vi "ROTPEN Control template CLEAN.vi"() -> ()   [LabVIEW 2018]
uses:
  <vilib>/Simulation/Scripting/Companion Diagram/SimConfigNode/SimParams.ctl
  <vilib>/Simulation/Scripting/Companion Diagram/SimConfigNode/_simSolvers.ctl
  <vilib>/Simulation/Implementation/Shared/SIMSCR Execution Mode.ctl
  <vilib>/Platform/TimedLoop/XDataNode/timing_clust.ctl
  <vilib>/Platform/TimedLoop/XDataNode/nitl_modes.ctl
  <vilib>/Platform/TimedLoop/XDataNode/wakeup.ctl
  <vilib>/Simulation/Param Hierarchy/Typedefs/SIMPH Param Control Actions.ctl
  <vilib>/addons/Control Design/_Stochastic Systems/Stochastic Systems.llb/Stochastic Systems SubVIs/cd_Second-Order Statistics Noise Model.ctl
  <vilib>/Simulation/Scripting/Editor Utilities/SIM subVI tag data.ctl
  <vilib>/Simulation/Scripting/Editor Utilities/SIM subVI execution type.ctl
  <vilib>/Simulation/Implementation/Shared/NILVSim_ParamChanged.vi
  <vilib>/Simulation/Implementation/Shared/NILVSim_FinishedLate.vi
  <vilib>/Simulation/Implementation/Shared/NILVSIM_BeginStep.vi
  <vilib>/Simulation/DataSources/Implementation/NILVSim Signal Generator.llb/SIM Signal Generator (scalar).vi
  <vilib>/Simulation/SignalArithmetic/Implementation/NILVSim Gain.llb/SIM Gain (scalar).vi
  <vilib>/Simulation/Utility/Implementation/SIM Halt.vi
  <vilib>/Simulation/ContinuousLinear/Implementation/NILVSim Derivative.llb/SIM derivative (scalar).vi
  <vilib>/Simulation/SignalArithmetic/Implementation/NILVSim Gain.llb/SIM Gain (vector,ScalarGain).vi
  <vilib>/Simulation/SignalArithmetic/Implementation/NILVSim Gain.llb/SIM Gain (dot product).vi
  <vilib>/Simulation/Nonlinear/Implementation/NILVSim Saturation.llb/SIM Saturation (scalar).vi
  <vilib>/Simulation/Implementation/Shared/SIM Fire Discrete SubVI.vi
  <vilib>/Simulation/Implementation/Shared/NILVSim_Manager.vi
  <vilib>/Utility/error.llb/Clear Errors.vi
  <vilib>/Simulation/Implementation/Shared/NILVSim_FinalizeModel.vi
  <vilib>/Simulation/Implementation/Shared/SIM Fire Discrete SubVI (Core).vi
  <vilib>/addons/Control Design/_Stochastic Systems/Stochastic Systems.llb/CD Construct Stochastic Model (Numeric).vi
  <vilib>/addons/Control Design/_Stochastic Systems/Stochastic Systems.llb/CD Construct Noise Model (Numeric).vi
  <vilib>/Simulation/Implementation/Shared/SIM Unbundle Sim Info.vi
  <vilib>/Simulation/Implementation/Shared/SIMSH Read Queue.vi
  <vilib>/Simulation/Implementation/Shared/NILVSim_Initialize.vi
  <vilib>/Simulation/Utility/Implementation/NILVSim Get Time and IsAcceptedStep.vi
  <vilib>/Simulation/Implementation/Shared/NILVSim_GetModelError.vi
  <vilib>/Simulation/Implementation/Shared/SIM Bundle Sim Info.vi
  <vilib>/Simulation/Scripting/Companion Diagram/SimConfigNode/SimDog.xnode
  <vilib>/Quanser/Rapid Control Prototyping Toolkit/hardware/HIL Immediate IO/_TypeSpecific/CL HIL Read Encoder (Vector).vi
  <vilib>/Quanser/Rapid Control Prototyping Toolkit/hardware/HIL Immediate IO/CL HIL Read.vi
  <vilib>/Quanser/Rapid Control Prototyping Toolkit/hardware/HIL Immediate IO/_TypeSpecific/CL HIL Write Analog (Scalar).vi
  <vilib>/Quanser/Rapid Control Prototyping Toolkit/hardware/HIL Immediate IO/CL HIL Write.vi
  <vilib>/addons/Control Design/_Implementation/CD Continuous Recursive Kalman Filter.vi
  <vilib>/Platform/TimedLoop/XDataNode/XDataNode.xnode
  <vilib>/Simulation/Implementation/XNodeFramework/SimXNode/SimX.xnode
  <vilib>/addons/Control Design/_Stochastic Systems/NI_CD_Stochastic Systems.lvlib
  <vilib>/Platform/TimedLoop/XDataNode/XDNodeRunTimeDep.lvlib
  <vilib>/Simulation/Implementation/Shared/NI_SIM_Implementation.lvlib
panel:
  out "Encoder Velocities (Kalman)":T1(graph)
  out "Encoder Angles (Kalman)":T1(graph)
  in  "stop":bool
  out "Motor Voltage (V)":dbl(graph)
  out "Encoder Angles (deg)":T2(graph)
  out "Encoder Velcoities (deg)":T3(graph)
  in  "Frequency (Hz)":dbl(slide)=0.2 min=0.0 max=0.5 step=0.05 scale=0.0..0.5 scale format="%#_3f"
  in  "Amplitude (deg)":dbl(slide) min=0.0 max=40.0 step=5.0 scale=0.0..40.0
  # "Rotary Arm Reference Signal"
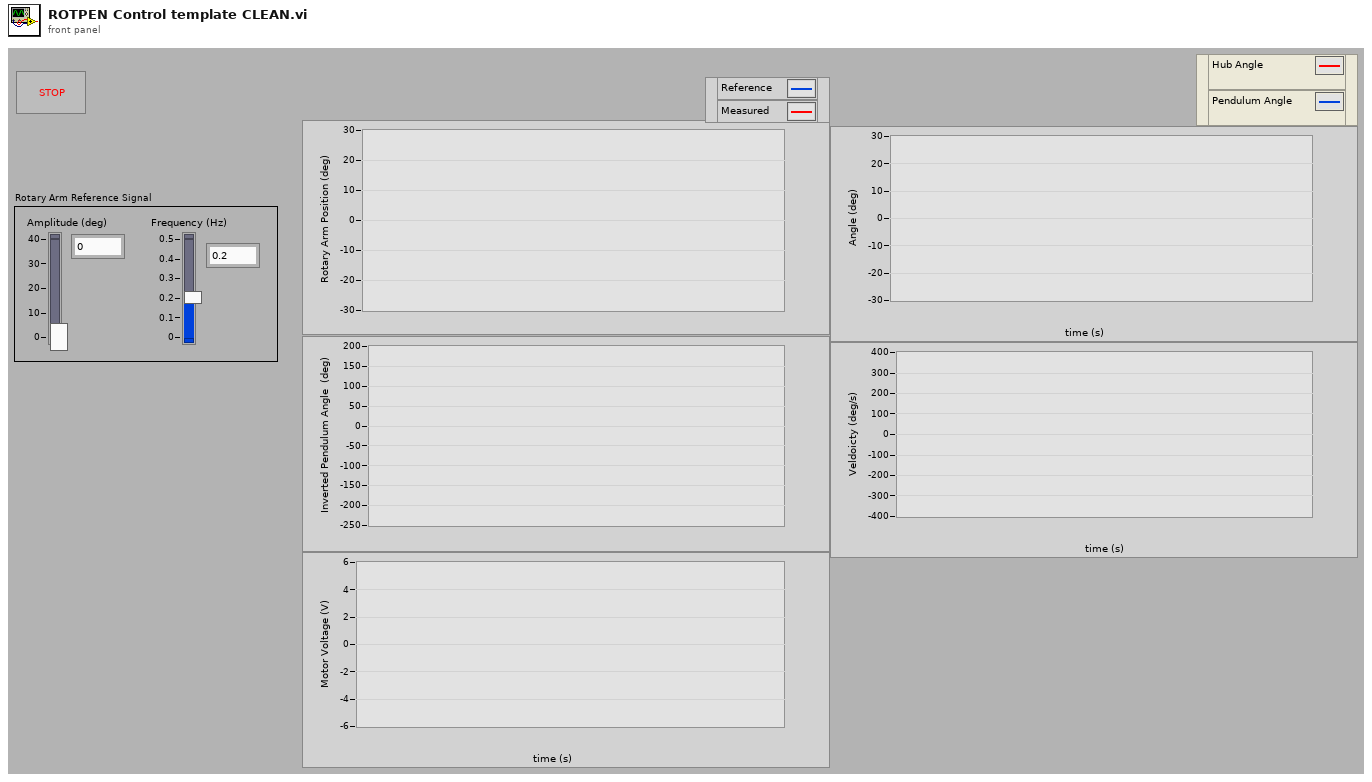
[diagram p1: front panel]
types:
  T1 = cluster{"Estimated State xhat(t)[0]":dbl, "Estimated State xhat(t)[1]":dbl, "Estimated State xhat(t)[2]":dbl, "Estimated State xhat(t)[3]":dbl, "Estimated State xhat(t)[4]":dbl, "Estimated State xhat(t)[5]":dbl, "Estimated State xhat(t)[6]":dbl, "Estimated State xhat(t)[7]":dbl, "Estimated State xhat(t)[8]":dbl}
  T2 = cluster{"output":dbl, "output":dbl, "output":dbl}
  T3 = cluster{"output[0]":dbl, "output[1]":dbl, "output[2]":dbl, "output[3]":dbl, "output[4]":dbl, "output[5]":dbl, "output[6]":dbl, "output[7]":dbl, "output[8]":dbl}
  T4 = typedef "NI_CD_Stochastic Systems.lvlib/cd_Stochastic State-Space Model.ctl" = cluster{"Sampling Time (s)":dbl, "G":dbl[][], "B":dbl[][], "A":dbl[][], "C":dbl[][], "D":dbl[][], "H":dbl[][]}
  T5 = typedef "NI_CD_Stochastic Systems.lvlib/cd_Second-Order Statistics Noise Model.ctl" = cluster{"Q":dbl[][], "E{w}":dbl[], "E{v}":dbl[], "R":dbl[][], "N":dbl[][]}
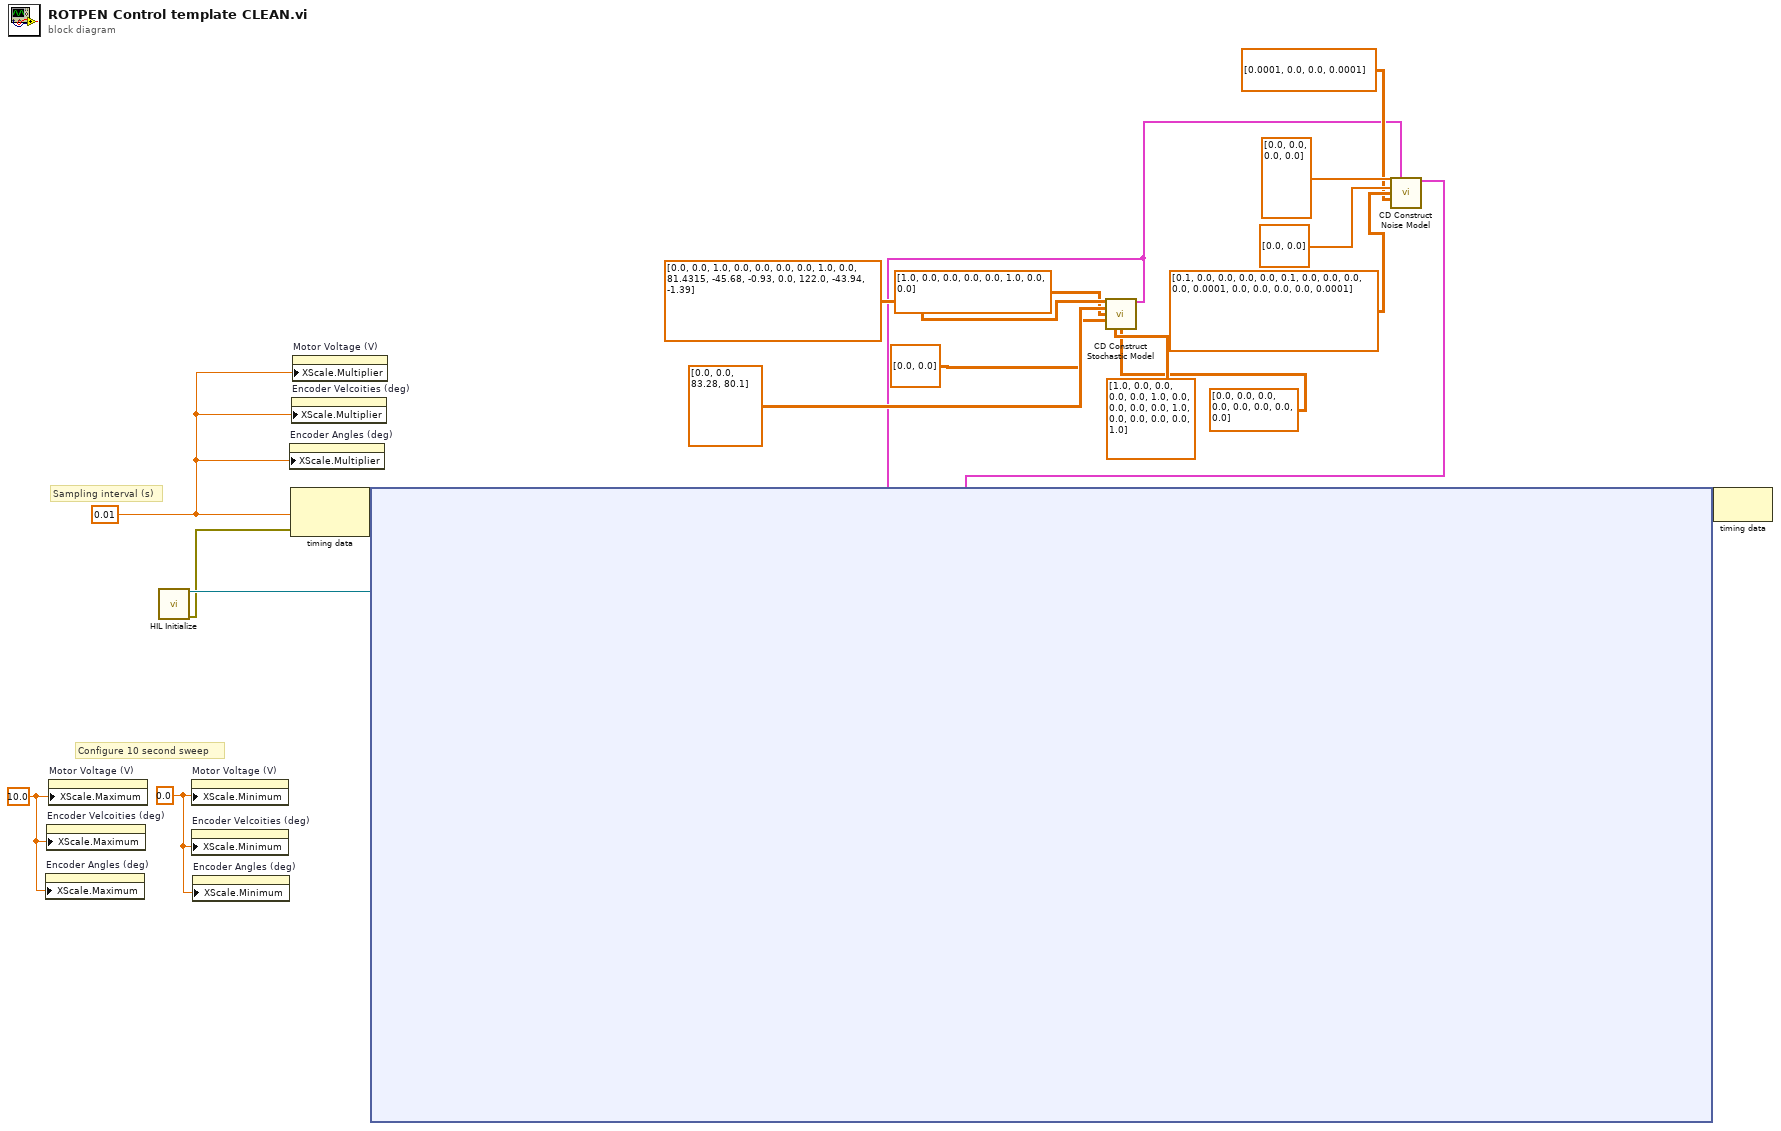
[diagram p0: block diagram]
diagram:
  w15 = 0.0 ("X Scale.Range:Maximum")
  w14 = 10.0 ("X Scale.Range:Maximum")
  w2 = 0.01 ("Step Size (s)")
  # "Configure 10 second sweep"
  # "Sampling interval (s)"
  n1 = property on="Encoder Angles (deg)" class="WFChart (strict)"("XScale.Maximum"=w14) -> ()  [unwired: 2 in, 2 out]
  n2 = property on="Encoder Velcoities (deg)" class="WFChart (strict)"("XScale.Maximum"=w14) -> ()  [unwired: 2 in, 2 out]
  n3 = property on="Motor Voltage (V)" class="WFChart (strict)"("XScale.Maximum"=w14) -> ()  [unwired: 2 in, 2 out]
  n4 = call "HIL Initialize"() -> ("board out"=w17:refnum<class "HIL Board.lvclass">, "error out"=w16:errorcluster)  [unwired: 14 in]
  n5 = property on="Motor Voltage (V)" class="WFChart (strict)"("XScale.Minimum"=w15) -> ()  [unwired: 2 in, 2 out]
  n6 = property on="Encoder Velcoities (deg)" class="WFChart (strict)"("XScale.Minimum"=w15) -> ()  [unwired: 2 in, 2 out]
  n7 = property on="Encoder Angles (deg)" class="WFChart (strict)"("XScale.Minimum"=w15) -> ()  [unwired: 2 in, 2 out]
  n8 = property on="Encoder Angles (deg)" class="WFChart (strict)"("XScale.Multiplier"=w2) -> ()  [unwired: 2 in, 2 out]
  n9 = node-c288(w2, w16) -> (w19:variant)
  n10 = property on="Encoder Velcoities (deg)" class="WFChart (strict)"("XScale.Multiplier"=w2) -> ()  [unwired: 2 in, 2 out]
  n11 = property on="Motor Voltage (V)" class="WFChart (strict)"("XScale.Multiplier"=w2) -> ()  [unwired: 2 in, 2 out]
  n12 = call-poly <vilib>:"CD Construct Stochastic Model.vi"("A"=dbl[][] [[0.0, 0.0, 1.0, 0.0], [0.0, 0.0, 0.0, 1.0], [0.0, 81.4315, -45.68, -0.93], [0.0, 122.0, -43.94, -1.39]], "B"=dbl[][] [[0.0], [0.0], [83.28], [80.1]], "C"=dbl[][] [[1.0, 0.0, 0.0, 0.0], [0.0, 1.0, 0.0, 0.0]], "D"=dbl[][] [[0.0], [0.0]], "G"=dbl[][] [[1.0, 0.0, 0.0, 0.0], [0.0, 1.0, 0.0, 0.0], [0.0, 0.0, 1.0, 0.0], [0.0, 0.0, 0.0, 1.0]], "H"=dbl[][] [[0.0, 0.0, 0.0, 0.0], [0.0, 0.0, 0.0, 0.0]]) -> ("Stochastic State-Space Model"=w4:T4)  [unwired: 8 in, 1 out]
  n13 = call-poly <vilib>:"CD Construct Noise Model.vi"("E{w}"=dbl[] [0.0, 0.0, 0.0, 0.0], "Stochastic State-Space Model"=w4, "E{v}"=dbl[] [0.0, 0.0], "Q"=dbl[][] [[0.1, 0.0, 0.0, 0.0], [0.0, 0.1, 0.0, 0.0], [0.0, 0.0, 0.0001, 0.0], [0.0, 0.0, 0.0, 0.0001]], "R"=dbl[][] [[0.0001, 0.0], [0.0, 0.0001]]) -> ("Second-Order Statistics Noise Model out"=w3:T5)  [unwired: 9 in, 1 out]
  n14 = node-c254 ("Control & Simulation Loop")(w19, w17, w4, w3) -> (w18:variant)
  n15 = node-c288(w18) -> ()  [unwired: 1 out]
